vi "Zernike_AE.vi"(7 "Action":enum16{"READ", "WRITE"}(ring), 10 "Zernike In":dbl[][][](array[numeric])) -> (2 "Zernike Out":dbl[][][](array[numeric]))   [LabVIEW 2014]
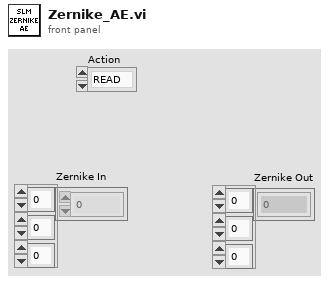
[diagram p1: front panel]
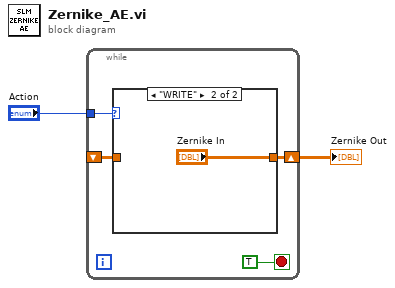
[diagram p0: block diagram]
diagram:
  n1 = while {
    tunnel: "Action" -> [w5]
    shift-right: [w4] -> w1
    shift-left: _ -> [w3]
    stop <- TRUE stop-if-true
    n2 = case shown="\"WRITE\"" w5 {
      tunnel: [w7 "Zernike In"] -> w4
      tunnel: w3 -> [w7 _]
      frame "READ", Default {
      }
      frame "WRITE" {
      }
    }
  }
  "Zernike Out" <- w1
